vi "Set Temperature.vi"(8 "error in (no error)":errorcluster, 10 "Setpoint":dbl, 11 "Huber Settings In":T1) -> (0 "error out":errorcluster, 1 "Connection Error":bool, 3 "Huber Settings Out":T1)   [LabVIEW 2021, in "Huber Ministat 230 TCU.lvlib"]
uses:
  Huber Ministat 230 TCU.lvlib
  Huber Settings.ctl
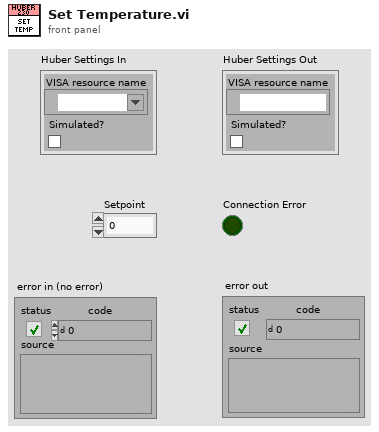
[diagram p1: front panel]
types:
  T1 = typedef "Huber Ministat 230 TCU.lvlib/Huber Settings.ctl" = cluster{"VISA resource name":refnum<visa-resource-name>, "Simulated?":bool}
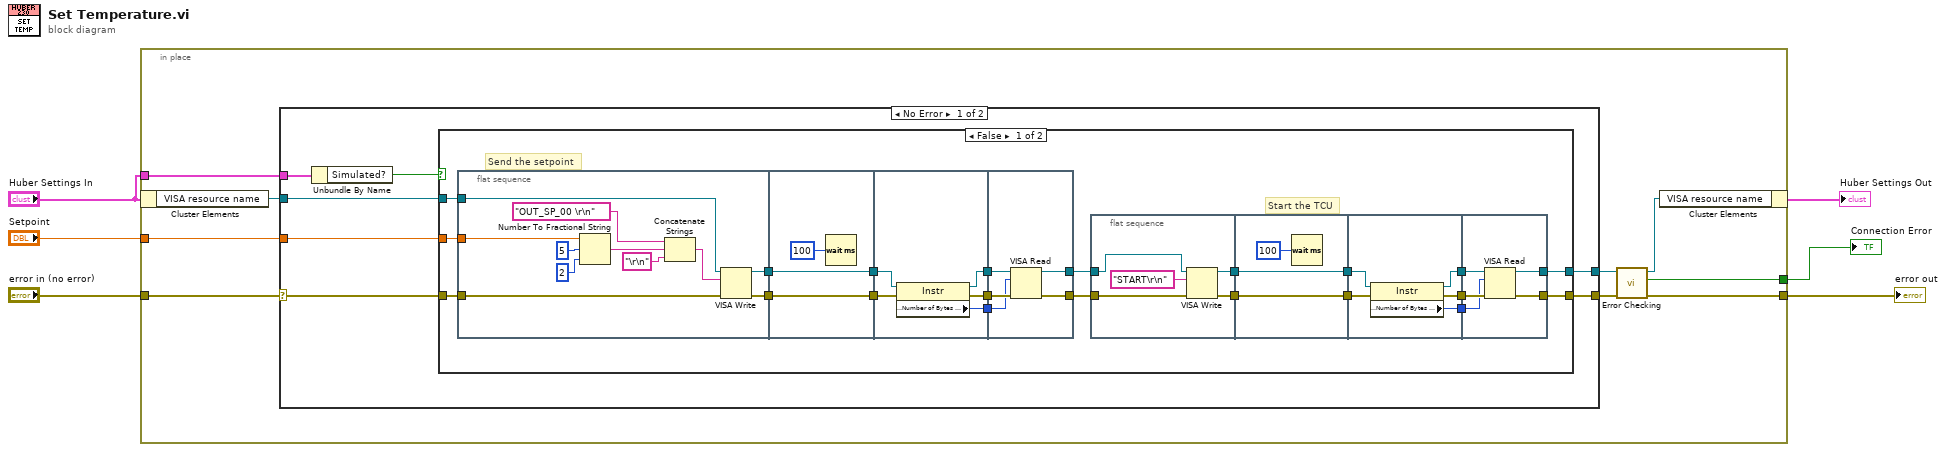
[diagram p0: block diagram]
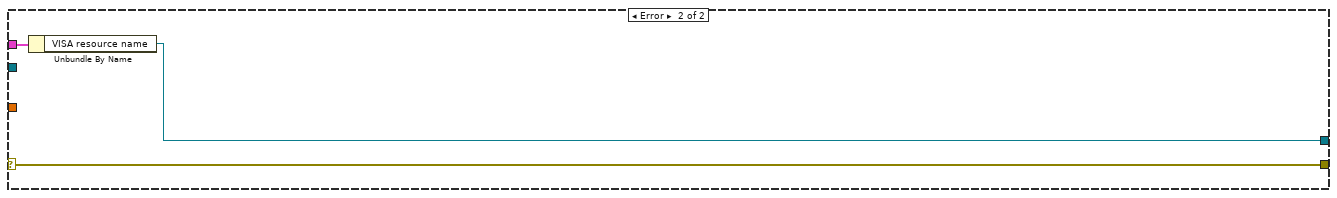
[diagram p3: hidden frame]
diagram:
  n1 = in-place {
    in-place-border: "error in (no error)" -> [w15]
    in-place-border: "Huber Settings In" -> [w12]
    in-place-border: "Setpoint" -> [w11]
    in-place-border: [w10] -> w4
    in-place-border: [w9] -> w3
    n2 = in-place-cluster #1("Huber Settings In") -> ("VISA resource name"=w8:refnum<visa-resource-name>)
    n3 = case shown="No Error" w15 {
      selector: w15 -> [w22 w90]
      tunnel: w12 -> [w18 w89]
      tunnel: [w21 w90] -> w13
      tunnel: [w20 w88] -> w14
      tunnel: w11 -> [w17 _]
      tunnel: w8 -> [w16 _]
      frame No Error {
        n4 = Unbundle By Name(w18) -> ("Simulated?"=w19:bool)
        n5 = case shown="False" w19 {
          tunnel: w22 -> [w42 w87]
          tunnel: [w24 w87] -> w21
          tunnel: [w25 w86] -> w20
          tunnel: w16 -> [w43 w86]
          tunnel: w17 -> [w23 _]
          frame False {
            # "Start the TCU"
            # "Send the setpoint"
            n6 = flat-sequence {
              tunnel: [w72] -> w41
              tunnel: [w71] -> w40
              tunnel: w43 -> [w70]
              tunnel: w42 -> [w69]
              tunnel: w23 -> [w65]
              tunnel: w41 -> [w74]
              tunnel: w40 -> [w73]
              tunnel: [w74] -> w39
              tunnel: [w73] -> w38
              tunnel: [w78] -> w37
              tunnel: [w77] -> w36
              tunnel: [w76] -> w35
              tunnel: w39 -> [w80]
              tunnel: w38 -> [w79]
              tunnel: [w85] -> w26
              tunnel: [w84] -> w27
              tunnel: w37 -> [w83]
              tunnel: w36 -> [w82]
              tunnel: w35 -> [w81]
              frame #0 {
                n7 = Number To Fractional String(number=w65, width (-)=i16 5, precision (6)=i16 2) -> (F-format string=w68:string)  [unwired: 1 in]
                n8 = Concatenate Strings("OUT_SP_00 \r\n" ("string"), w68, "\r\n" ("string")) -> (w62:string)
                n9 = VISA Write(VISA resource name=w70, write buffer=w62, error in (no error)=w69) -> (VISA resource name out=w72:refnum<visa-resource-name>, error out=w71:errorcluster)  [unwired: 1 out]
              }
              frame #1 {
                n10 = Wait (ms)(milliseconds to wait=u32 100) -> ()  [unwired: 1 out]
              }
              frame #2 {
                n11 = property class="Instr"(reference=w80, error in=w79) -> (reference out=w78:refnum<visa-resource-name>, error out=w77:errorcluster, "Serial Settings:Number of Bytes at Serial Port"=w76:u32)
              }
              frame #3 {
                n12 = VISA Read(VISA resource name=w83, byte count=w81, error in (no error)=w82) -> (VISA resource name out=w84:refnum<visa-resource-name>, error out=w85:errorcluster)  [unwired: 2 out]
              }
            }
            n13 = flat-sequence {
              tunnel: [w48] -> w34
              tunnel: [w47] -> w33
              tunnel: w27 -> [w46]
              tunnel: w26 -> [w45]
              tunnel: w34 -> [w50]
              tunnel: w33 -> [w49]
              tunnel: [w50] -> w32
              tunnel: [w49] -> w31
              tunnel: [w54] -> w30
              tunnel: [w53] -> w29
              tunnel: [w52] -> w28
              tunnel: w32 -> [w56]
              tunnel: w31 -> [w55]
              tunnel: [w61] -> w24
              tunnel: [w60] -> w25
              tunnel: w30 -> [w59]
              tunnel: w29 -> [w58]
              tunnel: w28 -> [w57]
              frame #0 {
                n14 = VISA Write(VISA resource name=w46, write buffer="START\r\n", error in (no error)=w45) -> (VISA resource name out=w48:refnum<visa-resource-name>, error out=w47:errorcluster)  [unwired: 1 out]
              }
              frame #1 {
                n15 = Wait (ms)(milliseconds to wait=u32 100) -> ()  [unwired: 1 out]
              }
              frame #2 {
                n16 = property class="Instr"(reference=w56, error in=w55) -> (reference out=w54:refnum<visa-resource-name>, error out=w53:errorcluster, "Serial Settings:Number of Bytes at Serial Port"=w52:u32)
              }
              frame #3 {
                n17 = VISA Read(VISA resource name=w59, byte count=w57, error in (no error)=w58) -> (VISA resource name out=w60:refnum<visa-resource-name>, error out=w61:errorcluster)  [unwired: 2 out]
              }
            }
          }
          frame True {
          }
        }
      }
      frame Error {
        n18 = Unbundle By Name(w89) -> ("VISA resource name"=w88:refnum<visa-resource-name>)
      }
    }
    n19 = call "Error Checking.vi"("error in (no error)"=w13, "VISA resource name"=w14) -> ("error out"=w9:errorcluster, "Connection Error"=w10:bool, "VISA resource name"=w7:refnum<visa-resource-name>)  [unwired: 7 in]
    n20 = in-place-cluster #1("VISA resource name"=w7) -> (→"Huber Settings Out":T1)
  }
  "error out" <- w3
  "Connection Error" <- w4
